vi "sv_Convert to Nominal Frequency.vi"(0 "bandwidth":T1(ring)=enum."1/3 octave", 2 "octave band selector":i32, 3 "midband frequency [Hz]":dbl format="%.2f", 4 "include units (T)":bool=TRUE) -> (5 "nominal frequency [Hz]":dbl format="%.2f", 6 "nominal frequency (string)":string)   [LabVIEW 2017, in "SoundVib_Octave_2014 standard.lvlib"]
uses:
  <vilib>/addons/Sound and Vibration/svt_Octave/SoundVib_Octave_2014 standard.lvlib
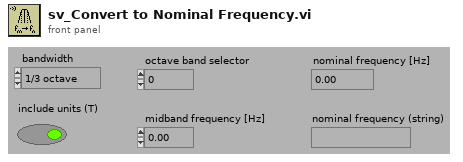
[diagram p1: front panel]
types:
  T1 = enum16{"1 octave", "1/3 octave", "1/6 octave", "1/12 octave", "1/24 octave", "1/48 octave", "1/96 octave"}
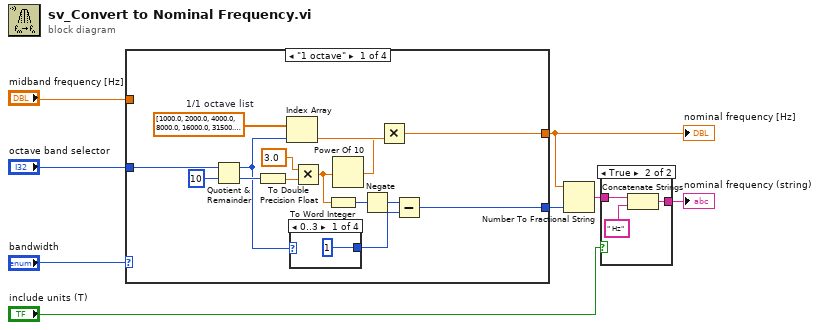
[diagram p0: block diagram]
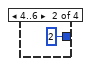
[diagram p3: hidden frame]
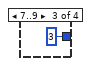
[diagram p4: hidden frame]
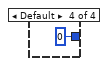
[diagram p5: hidden frame]
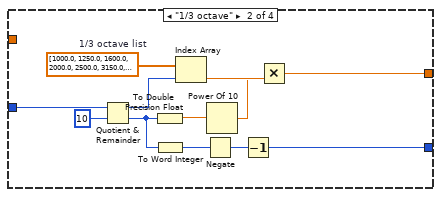
[diagram p6: hidden frame]
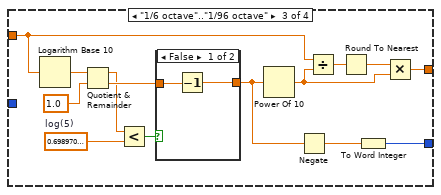
[diagram p7: hidden frame]
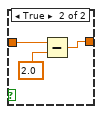
[diagram p8: hidden frame]
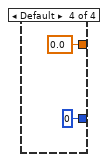
[diagram p9: hidden frame]
diagram:
  n1 = case shown="\"1 octave\"" "bandwidth" {
    tunnel: "octave band selector" -> [w23 w39 _ _]
    tunnel: [w19 w34 w43 0.0] -> w5
    tunnel: [w12 w30 w40 i16 0] -> w3
    tunnel: "midband frequency [Hz]" -> [_ _ w41 _]
    frame "1 octave" {
      w9 = dbl[] [1000.0, 2000.0, 4000.0, 8000.0, 16000.0, 31500.0, 63000.0, 125000.0, 250000.0, 500000.0]  # 1/1 octave list
      n2 = Quotient & Remainder(x=w23, y=10) -> (x-y*floor(x/y)=w14:i32, floor(x/y)=w16:i32)
      n3 = To Double Precision Float(number=w16) -> (double precision float=w18:dbl)
      n4 = Index Array(array=w9, index=w14) -> (element=w21:dbl)
      n5 = case shown="0..3" w14 {
        tunnel: [i16 1 ("y") i16 2 ("y") i16 3 ("y") i16 0 ("y")] -> w10
        frame 0..3 {
        }
        frame 4..6 {
        }
        frame 7..9 {
        }
        frame Default {
        }
      }
      n6 = Multiply(x=3.0 ("y"), y=w18) -> (x*y=w15:dbl)
      n7 = To Word Integer(number=w15) -> (16bit integer=w13:i16)
      n8 = Power Of 10(x=w15) -> (10^x=w20:dbl)
      n9 = Negate(x=w13) -> (-x=w11:i16)
      n10 = Multiply(x=w21, y=w20) -> (x*y=w19:dbl)
      n11 = Subtract(x=w11, y=w10) -> (x-y=w12:i16)
    }
    frame "1/3 octave" {
      w28 = dbl[] [1000.0, 1250.0, 1600.0, 2000.0, 2500.0, 3150.0, 4000.0, 5000.0, 6300.0, 8000.0]  # 1/3 octave list
      n12 = Quotient & Remainder(x=w39, y=10) -> (x-y*floor(x/y)=w37:i32, floor(x/y)=w31:i32)
      n13 = To Double Precision Float(number=w31) -> (double precision float=w33:dbl)
      n14 = To Word Integer(number=w31) -> (16bit integer=w29:i16)
      n15 = Index Array(array=w28, index=w37) -> (element=w36:dbl)
      n16 = Negate(x=w29) -> (-x=w32:i16)
      n17 = Power Of 10(x=w33) -> (10^x=w35:dbl)
      n18 = Decrement(x=w32) -> (x-1=w30:i16)
      n19 = Multiply(x=w36, y=w35) -> (x*y=w34:dbl)
    }
    frame "1/6 octave".."1/96 octave" {
      w45 = 0.6989700043360189  # log(5)
      n20 = Logarithm Base 10(1:w41) -> (0:w50:dbl)
      n21 = Quotient & Remainder(x=w50, y=1.0) -> (x-y*floor(x/y)=w47:dbl, floor(x/y)=w48:dbl)
      n22 = Less?(x=w47, y=w45) -> (x < y?=w46:bool)
      n23 = case shown="False" w46 {
        tunnel: w48 -> [w55 w57]
        tunnel: [w54 w58] -> w44
        frame False {
          n24 = Decrement(x=w55) -> (x-1=w54:dbl)
        }
        frame True {
          n25 = Subtract(x=w57, y=2.0) -> (x-y=w58:dbl)
        }
      }
      n26 = Power Of 10(x=w44) -> (10^x=w51:dbl)
      n27 = Negate(x=w44) -> (-x=w42:dbl)
      n28 = Divide(x=w41, y=w51) -> (x/y=w53:dbl)
      n29 = Round To Nearest(number=w53) -> (nearest integer value=w52:dbl)
      n30 = To Word Integer(number=w42) -> (16bit integer=w40:i16)
      n31 = Multiply(x=w52, y=w51) -> (x*y=w43:dbl)
    }
    frame Default {
    }
  }
  "nominal frequency [Hz]" <- w5
  n32 = Number To Fractional String(number=w5, precision (6)=w3) -> (F-format string=w6:string)  [unwired: 2 in]
  n33 = case shown="True" "include units (T)" {
    tunnel: w6 -> [w61 w63]
    tunnel: [w61 w62] -> w4
    frame False {
    }
    frame True {
      n34 = Concatenate Strings(w63, " Hz") -> (w62:string)
    }
  }
  "nominal frequency (string)" <- w4
